vi "Finish.vi"   [LabVIEW 2014]
doc: "This VI is called just before exiting. It is expected to close I/O refnum, save collected data, etc."
uses:
  <vilib>/Rock Robotics/WPI/Joystick/WPI_JoystickGetSetRefNum.vi
  <vilib>/Rock Robotics/WPI/RobotDrive/WPI_RobotDriveGetSetRefNum.vi
  <vilib>/Rock Robotics/WPI/Compressor/WPI_CompressorGetSetRefNum.vi
types:
  T1 = typedef "WPI_RobotDriveDevRef.ctl" = cluster{"DevStatus":errorcluster, "Motors[]":T2[], "Square Inputs":bool, "Max Output":dbl}
  T2 = typedef "WPI_MotorControlDeviceRef.ctl" = cluster{"DeviceStatus":errorcluster, "Type":T3, "PWM":cluster{"Controller":T4, "PWM Channel":T5, "DeadBand":T6}, "CAN":cluster{"Device Number":u8, "Control Mode":T7, "Semaphore":T8, "Max Vout":dbl, "TalonSRX Control Mode":T9}, "Invert":bool, "TransformRef":T10, "InvTransformRef":T10}
  T3 = typedef "WPI_MotorControlType.ctl" = enum16{"PWM", "CAN", "CANTalonSRX"}
  T4 = typedef "FPGA_TypedefDigitalModule.ctl" = enum16{"Controller 1"}
  T5 = typedef "FPGA_DIOPWMChannel.ctl" = enum8{"PWM 0", "PWM 1", "PWM 2", "PWM 3", "PWM 4", "PWM 5", "PWM 6", "PWM 7", "PWM 8", "PWM 9", "PWM MXP 0", "PWM MXP 1", "PWM MXP 2", "PWM MXP 3", "PWM MXP 4", "PWM MXP 5", "PWM MXP 6", "PWM MXP 7", "PWM MXP 8", "PWM MXP 9", "Invalid"}
  T6 = typedef "WPI_PWMDeadband.ctl" = cluster{"Name":string, "maxPositivePwm":i32, "minPositivePwm":i32, "centerPwm":i32, "maxNegativePwm":i32, "minNegativePwm":i32, "angularRange":u16}
  T7 = typedef "WPI_CANJaguar_ControlMode.ctl" = enum8{"Percent VBus", "Current", "Speed", "Position", "Voltage"}
  T8 = typedef "Semaphore RefNum" = refnum<k1>
  T9 = typedef "WPI_CANTalonSRX_APIControlMode.ctl" = enum8{"Percent VBus", "Speed", "Position", "Slave", "Unchanged / Invalid"}
  T10 = typedef "WPI_PWMTransform_ConPane.ctl" = refnum<vi>
  T11 = typedef "WPI_EncoderDevRef.ctl" = cluster{"DevStatus":errorcluster, "EncoderIndex":T12, "CounterIndex":T13, "DistancePerCount":dbl, "Decoding Type":T14}
  T12 = typedef "FPGA_EncoderIdx.ctl" = enum8{"Enc 0", "Enc 1", "Enc 2", "Enc 3", "Enc 4", "Enc 5", "Enc 6", "Enc 7", "Invalid"}
  T13 = typedef "FPGA_CounterCtrSystemIndex.ctl" = enum8{"Ctr 0", "Ctr 1", "Ctr 2", "Ctr 3", "Ctr 4", "Ctr 5", "Ctr 6", "Ctr 7", "Invalid"}
  T14 = typedef "WPI_EncoderType.ctl" = enum16{"1x", "2x", "4x"}
  T15 = typedef "WPI_DigitalInputDevRef.ctl" = cluster{"DevStatus":errorcluster, "DIO Channel":T16, "Controller":T4}
  T16 = typedef "FPGA_DIOChannel.ctl" = enum8{"DIO 0", "DIO 1", "DIO 2", "DIO 3", "DIO 4", "DIO 5", "DIO 6", "DIO 7", "DIO 8", "DIO 9", "DIO MXP 0", "DIO MXP 1", "DIO MXP 2", "DIO MXP 3", "DIO MXP 4", "DIO MXP 5", "DIO MXP 6", "DIO MXP 7", "DIO MXP 8", "DIO MXP 9", "DIO MXP 10", "DIO MXP 11", "DIO MXP 12", "DIO MXP 13", "DIO MXP 14", "DIO MXP 15", "Invalid"}
  T17 = typedef "WPI_JoystickDevRef.ctl" = cluster{"Device":T18}
  T18 = typedef "WPI_JoystickDeviceEnum.ctl" = enum16{"USB 0", "USB 1", "USB 2", "USB 3", "USB 4", "USB 5"}
  T19 = typedef "WPI_CompressorDevRef.ctl" = cluster{"DevStatus":errorcluster, "Pneumatics Control Module":u8}
  T20 = typedef "WPI_SolenoidDevRef.ctl" = cluster{"DevStatus":errorcluster, "Pneumatics Control Module":u8, "Forward Solenoid Channel":T21, "Reverse Solenoid Channel":T21}
  T21 = typedef "WPI_SolenoidChannel.ctl" = enum8{"Solenoid 0", "Solenoid 1", "Solenoid 2", "Solenoid 3", "Solenoid 4", "Solenoid 5", "Solenoid 6", "Solenoid 7", "Invalid"}
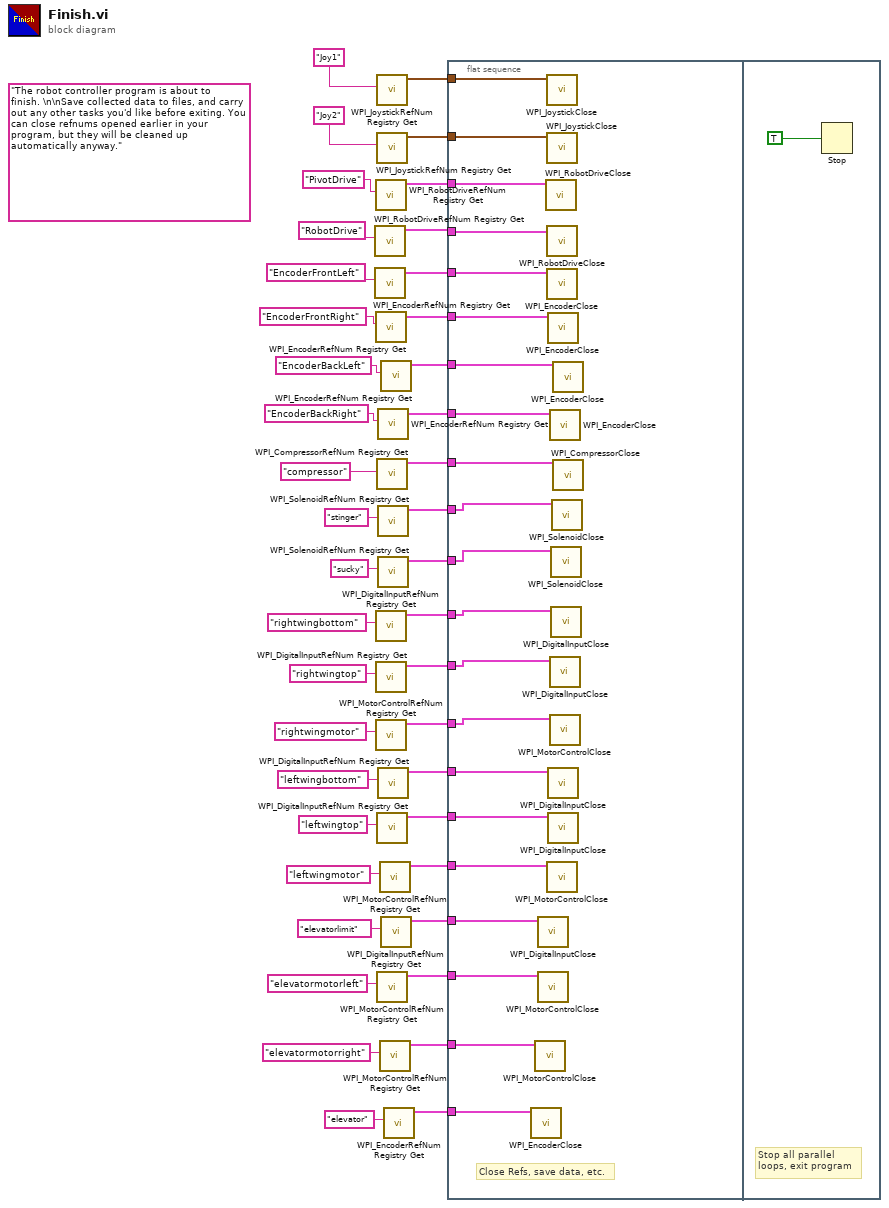
[diagram p0: block diagram]
diagram:
  (unwired) "The robot controller program is about to finish. \n\nSave collected data to files, and carry out any other tasks you'd like before exiting. You can close refnums opened earlier in your program, but they will be cleaned up automatically anyway."
  n1 = call <vilib>:"WPI_RobotDriveRefNum Registry Get.vi"("refnum name"="RobotDrive") -> ("RobotDriveDevRef"=w38:T1)  [unwired: 9 in, 1 out]
  n2 = call <vilib>:"WPI_EncoderRefNum Registry Get.vi"("refnum name"="EncoderFrontLeft") -> ("EncoderDevRef"=w33:T11)  [unwired: 9 in, 1 out]
  n3 = call <vilib>:"WPI_RobotDriveRefNum Registry Get.vi"("refnum name"="PivotDrive") -> ("RobotDriveDevRef"=w40:T1)  [unwired: 1 in, 9 out]
  n4 = call <vilib>:"WPI_EncoderRefNum Registry Get.vi"("refnum name"="EncoderFrontRight") -> ("EncoderDevRef"=w27:T11)  [unwired: 9 in, 1 out]
  n5 = call <vilib>:"WPI_DigitalInputRefNum Registry Get.vi"("refnum name"="rightwingbottom") -> ("DigitalInputDevRef"=w18:T15)  [unwired: 9 in, 1 out]
  n6 = call <vilib>:"WPI_DigitalInputRefNum Registry Get.vi"("refnum name"="rightwingtop") -> ("DigitalInputDevRef"=w17:T15)  [unwired: 9 in, 1 out]
  n7 = call <vilib>:"WPI_MotorControlRefNum Registry Get.vi"("refnum name"="rightwingmotor") -> ("MotorControlDevRef"=w15:T2)  [unwired: 9 in, 1 out]
  n8 = call <vilib>:"WPI_JoystickRefNum Registry Get.vi"("refnum name"="Joy1") -> ("JoystickDevRef"=w36:T17)  [unwired: 1 in, 9 out]
  n9 = call <vilib>:"WPI_JoystickRefNum Registry Get.vi"("refnum name"="Joy2") -> ("JoystickDevRef"=w39:T17)  [unwired: 1 in, 9 out]
  n10 = call <vilib>:"WPI_CompressorRefNum Registry Get.vi"("refnum name"="compressor") -> ("CompressorDevRef"=w25:T19)  [unwired: 9 in, 1 out]
  n11 = call <vilib>:"WPI_DigitalInputRefNum Registry Get.vi"("refnum name"="leftwingtop") -> ("DigitalInputDevRef"=w12:T15)  [unwired: 9 in, 1 out]
  n12 = call <vilib>:"WPI_MotorControlRefNum Registry Get.vi"("refnum name"="elevatormotorleft") -> ("MotorControlDevRef"=w8:T2)  [unwired: 9 in, 1 out]
  n13 = call <vilib>:"WPI_EncoderRefNum Registry Get.vi"("refnum name"="EncoderBackRight") -> ("EncoderDevRef"=w29:T11)  [unwired: 9 in, 1 out]
  n14 = call <vilib>:"WPI_SolenoidRefNum Registry Get.vi"("refnum name"="stinger") -> ("SolenoidDevRef"=w23:T20)  [unwired: 9 in, 1 out]
  n15 = call <vilib>:"WPI_SolenoidRefNum Registry Get.vi"("refnum name"="sucky") -> ("SolenoidDevRef"=w21:T20)  [unwired: 9 in, 1 out]
  n16 = call <vilib>:"WPI_DigitalInputRefNum Registry Get.vi"("refnum name"="leftwingbottom") -> ("DigitalInputDevRef"=w14:T15)  [unwired: 9 in, 1 out]
  n17 = call <vilib>:"WPI_MotorControlRefNum Registry Get.vi"("refnum name"="leftwingmotor") -> ("MotorControlDevRef"=w10:T2)  [unwired: 9 in, 1 out]
  n18 = call <vilib>:"WPI_MotorControlRefNum Registry Get.vi"("refnum name"="elevatormotorright") -> ("MotorControlDevRef"=w6:T2)  [unwired: 9 in, 1 out]
  n19 = call <vilib>:"WPI_EncoderRefNum Registry Get.vi"("refnum name"="EncoderBackLeft") -> ("EncoderDevRef"=w28:T11)  [unwired: 9 in, 1 out]
  n20 = call <vilib>:"WPI_DigitalInputRefNum Registry Get.vi"("refnum name"="elevatorlimit") -> ("DigitalInputDevRef"=w7:T15)  [unwired: 9 in, 1 out]
  n21 = call <vilib>:"WPI_EncoderRefNum Registry Get.vi"("refnum name"="elevator") -> ("EncoderDevRef"=w2:T11)  [unwired: 9 in, 1 out]
  n22 = flat-sequence {
    tunnel: w40 -> [w63]
    tunnel: w39 -> [w62]
    tunnel: w38 -> [w61]
    tunnel: w36 -> [w60]
    tunnel: w33 -> [w59]
    tunnel: w29 -> [w58]
    tunnel: w28 -> [w57]
    tunnel: w27 -> [w56]
    tunnel: w25 -> [w55]
    tunnel: w23 -> [w54]
    tunnel: w21 -> [w53]
    tunnel: w18 -> [w52]
    tunnel: w17 -> [w51]
    tunnel: w15 -> [w50]
    tunnel: w14 -> [w49]
    tunnel: w12 -> [w48]
    tunnel: w10 -> [w47]
    tunnel: w8 -> [w46]
    tunnel: w7 -> [w45]
    tunnel: w6 -> [w44]
    tunnel: w2 -> [w43]
    frame #0 {
      # "Close Refs, save data, etc."
      n23 = call <vilib>:"WPI_EncoderClose.vi"("EncoderDevRef"=w43) -> ()  [unwired: 10 in, 1 out]
      n24 = call <vilib>:"WPI_MotorControlClose.vi"("MotorControlDevRef"=w44) -> ()  [unwired: 10 in, 1 out]
      n25 = call <vilib>:"WPI_DigitalInputClose.vi"("DigitalInputDevRef"=w45) -> ()  [unwired: 10 in, 1 out]
      n26 = call <vilib>:"WPI_MotorControlClose.vi"("MotorControlDevRef"=w46) -> ()  [unwired: 10 in, 1 out]
      n27 = call <vilib>:"WPI_RobotDriveClose.vi"("RobotDriveDevRef"=w63) -> ()  [unwired: 1 in, 10 out]
      n28 = call <vilib>:"WPI_JoystickClose.vi"("JoystickDevRef"=w60) -> ()  [unwired: 11 out]
      n29 = call <vilib>:"WPI_JoystickClose.vi"("JoystickDevRef"=w62) -> ()  [unwired: 11 out]
      n30 = call <vilib>:"WPI_RobotDriveClose.vi"("RobotDriveDevRef"=w61) -> ()  [unwired: 1 in, 10 out]
      n31 = call <vilib>:"WPI_EncoderClose.vi"("EncoderDevRef"=w59) -> ()  [unwired: 10 in, 1 out]
      n32 = call <vilib>:"WPI_MotorControlClose.vi"("MotorControlDevRef"=w47) -> ()  [unwired: 10 in, 1 out]
      n33 = call <vilib>:"WPI_EncoderClose.vi"("EncoderDevRef"=w56) -> ()  [unwired: 10 in, 1 out]
      n34 = call <vilib>:"WPI_DigitalInputClose.vi"("DigitalInputDevRef"=w49) -> ()  [unwired: 10 in, 1 out]
      n35 = call <vilib>:"WPI_DigitalInputClose.vi"("DigitalInputDevRef"=w48) -> ()  [unwired: 10 in, 1 out]
      n36 = call <vilib>:"WPI_EncoderClose.vi"("EncoderDevRef"=w58) -> ()  [unwired: 10 in, 1 out]
      n37 = call <vilib>:"WPI_DigitalInputClose.vi"("DigitalInputDevRef"=w51) -> ()  [unwired: 10 in, 1 out]
      n38 = call <vilib>:"WPI_MotorControlClose.vi"("MotorControlDevRef"=w50) -> ()  [unwired: 10 in, 1 out]
      n39 = call <vilib>:"WPI_SolenoidClose.vi"("SolenoidDevRef"=w53) -> ()  [unwired: 10 in, 1 out]
      n40 = call <vilib>:"WPI_DigitalInputClose.vi"("DigitalInputDevRef"=w52) -> ()  [unwired: 10 in, 1 out]
      n41 = call <vilib>:"WPI_SolenoidClose.vi"("SolenoidDevRef"=w54) -> ()  [unwired: 10 in, 1 out]
      n42 = call <vilib>:"WPI_EncoderClose.vi"("EncoderDevRef"=w57) -> ()  [unwired: 10 in, 1 out]
      n43 = call <vilib>:"WPI_CompressorClose.vi"("CompressorDevRef"=w55) -> ()  [unwired: 10 in, 1 out]
    }
    frame #1 {
      # "Stop all parallel\nloops, exit program"
      n44 = Stop(stop? (T)=TRUE ("Quit")) -> ()
    }
  }
